vi "Write Binary Address.vi"(8 "error in (no error)":errorcluster, 10 "Binary Address":i16[](array[numeric]), 11 "Addressing Mode in":refnum<class "Addressing Mode.lvclass">) -> (0 "error out":errorcluster, 3 "Addressing Mode out":refnum<class "Addressing Mode.lvclass">)   [LabVIEW 2020, in "Addressing Mode.lvclass"]
uses:
  Addressing Mode.lvclass
  Addressing Mode.lvclass/Addressing Mode.ctl
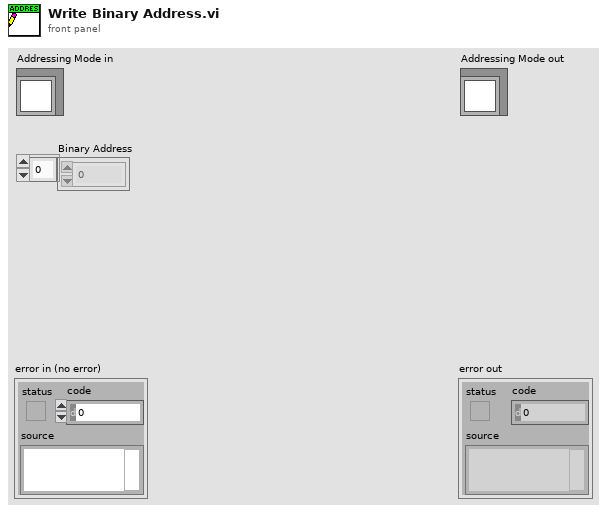
[diagram p1: front panel]
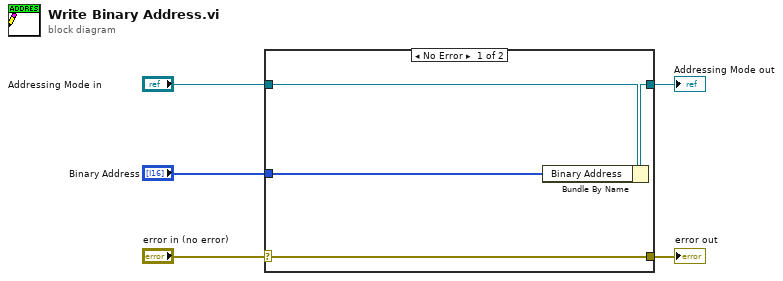
[diagram p0: block diagram]
diagram:
  n1 = case shown="No Error" "error in (no error)" {
    selector: "error in (no error)" -> [w9 w10]
    tunnel: [w9 w10] -> w4
    tunnel: [w7 w11] -> w2
    tunnel: "Addressing Mode in" -> [w8 w11]
    tunnel: "Binary Address" -> [w6 _]
    frame No Error {
      n2 = Bundle By Name(cluster=w8, "Binary Address"=w6) -> (w7:refnum<class "Addressing Mode.lvclass">)
    }
    frame Error {
    }
  }
  "error out" <- w4
  "Addressing Mode out" <- w2
